vi "Begin.vi"(8 "error in":errorcluster) -> (0 "error out":errorcluster)   [LabVIEW 2014]
doc: "Called before other user functions, this VI is expected to open initial I/O refnums, load in file data, and do all program initialization. Notice that the <B>error out</B> terminal is simply used for data flow. Wiring it to other structures or subVIs ensures that this VI runs first."
uses:
  <vilib>/Rock Robotics/WPI/DriverStation/WPI_DriverStationRobotMode2.ctl
  <vilib>/Rock Robotics/WPI/Joystick/WPI_JoystickDeviceEnum.ctl
  <vilib>/Rock Robotics/SystemInterfaces/DIO/FPGA_DIOPWMChannel.ctl
  <vilib>/Rock Robotics/WPI/Accelerometer/WPI_AccelerometerRange.ctl
  <vilib>/Rock Robotics/SystemInterfaces/AI/FPGA_AIGyroChannel.ctl
  <vilib>/Rock Robotics/WPI/Solenoid/WPI_SolenoidChannel.ctl
  <vilib>/Rock Robotics/SystemInterfaces/DIO/FPGA_DIOChannel.ctl
  <vilib>/Rock Robotics/WPI/Encoder/WPI_EncoderType.ctl
  <vilib>/Rock Robotics/SystemInterfaces/DIO/FPGA_DIORelayChannel.ctl
  Support Files/Robot Global Data.vi
  <vilib>/Rock Robotics/Network Tables/SD Write String Array.vi
  <vilib>/Rock Robotics/WPI/MotorControl/WPI_MotorControlOpen Talon.vi
  <vilib>/Rock Robotics/WPI/Accelerometer/InternalAccelerometer/WPI_AccelerometerInternalOpen.vi
  <vilib>/Rock Robotics/WPI/Solenoid/WPI_SolenoidOpenDouble.vi
  <vilib>/Rock Robotics/WPI/Counter/WPI_CounterDigitalInputToDigitalSource.vi
  <vilib>/Rock Robotics/WPI/Switch/WPI_SwitchOpenLimit.vi
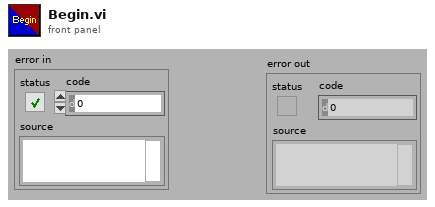
[diagram p1: front panel]
types:
  T1 = typedef "FPGA_DIORelayChannel.ctl" = enum8{"Relay 0", "Relay 1", "Relay 2", "Relay 3", "Invalid"}
  T2 = typedef "FPGA_DIOChannel.ctl" = enum8{"DIO 0", "DIO 1", "DIO 2", "DIO 3", "DIO 4", "DIO 5", "DIO 6", "DIO 7", "DIO 8", "DIO 9", "DIO MXP 0", "DIO MXP 1", "DIO MXP 2", "DIO MXP 3", "DIO MXP 4", "DIO MXP 5", "DIO MXP 6", "DIO MXP 7", "DIO MXP 8", "DIO MXP 9", "DIO MXP 10", "DIO MXP 11", "DIO MXP 12", "DIO MXP 13", "DIO MXP 14", "DIO MXP 15", "Invalid"}
  T3 = typedef "WPI_EncoderType.ctl" = enum16{"1x", "2x", "4x"}
  T4 = typedef "WPI_SolenoidChannel.ctl" = enum8{"Solenoid 0", "Solenoid 1", "Solenoid 2", "Solenoid 3", "Solenoid 4", "Solenoid 5", "Solenoid 6", "Solenoid 7", "Invalid"}
  T5 = typedef "FPGA_DIOPWMChannel.ctl" = enum8{"PWM 0", "PWM 1", "PWM 2", "PWM 3", "PWM 4", "PWM 5", "PWM 6", "PWM 7", "PWM 8", "PWM 9", "PWM MXP 0", "PWM MXP 1", "PWM MXP 2", "PWM MXP 3", "PWM MXP 4", "PWM MXP 5", "PWM MXP 6", "PWM MXP 7", "PWM MXP 8", "PWM MXP 9", "Invalid"}
  T6 = typedef "FPGA_AIGyroChannel.ctl" = enum8{"AI 0", "AI 1", "Invalid"}
  T7 = typedef "WPI_AccelerometerRange.ctl" = enum16{"+/- 2 g", "+/- 4 g", "+/- 8 g"}
  T8 = typedef "WPI_JoystickDeviceEnum.ctl" = enum16{"USB 0", "USB 1", "USB 2", "USB 3", "USB 4", "USB 5"}
  T9 = typedef "WPI_DriverStationRobotMode2.ctl" = enum16{"Autonomous Disabled", "Autonomous Enabled", "Teleop Disabled", "Teleop Enabled", "Disconnected", "Finish", "Test Disabled", "Test Enabled", "Emergency Stopped"}
  T10 = typedef "WPI_JoystickDevRef.ctl" = cluster{"Device":T8}
  T11 = typedef "WPI_SwitchDevRef.ctl" = cluster{"DevStatus":errorcluster, "DIO Channel":T2, "Controller":T12, "CntIndex":T13, "Normally Closed":bool}
  T12 = typedef "FPGA_TypedefDigitalModule.ctl" = enum16{"Controller 1"}
  T13 = typedef "FPGA_CounterCtrSystemIndex.ctl" = enum8{"Ctr 0", "Ctr 1", "Ctr 2", "Ctr 3", "Ctr 4", "Ctr 5", "Ctr 6", "Ctr 7", "Invalid"}
  T14 = typedef "WPI_RelayDevRef.ctl" = cluster{"DevStatus":errorcluster, "Relay Channel":T1, "Controller":T12, "Relay Direction":T15}
  T15 = typedef "WPI_RelayDirection.ctl" = enum16{"Both directions", "Forward only", "Reverse only"}
  T16 = typedef "WPI_MotorControlDeviceRef.ctl" = cluster{"DeviceStatus":errorcluster, "Type":T17, "PWM":cluster{"Controller":T12, "PWM Channel":T5, "DeadBand":T18}, "CAN":cluster{"Device Number":u8, "Control Mode":T19, "Semaphore":T20, "Max Vout":dbl, "TalonSRX Control Mode":T21}, "Invert":bool, "TransformRef":T22, "InvTransformRef":T22}
  T17 = typedef "WPI_MotorControlType.ctl" = enum16{"PWM", "CAN", "CANTalonSRX"}
  T18 = typedef "WPI_PWMDeadband.ctl" = cluster{"Name":string, "maxPositivePwm":i32, "minPositivePwm":i32, "centerPwm":i32, "maxNegativePwm":i32, "minNegativePwm":i32, "angularRange":u16}
  T19 = typedef "WPI_CANJaguar_ControlMode.ctl" = enum8{"Percent VBus", "Current", "Speed", "Position", "Voltage"}
  T20 = typedef "Semaphore RefNum" = refnum<k1>
  T21 = typedef "WPI_CANTalonSRX_APIControlMode.ctl" = enum8{"Percent VBus", "Speed", "Position", "Slave", "Unchanged / Invalid"}
  T22 = typedef "WPI_PWMTransform_ConPane.ctl" = refnum<vi>
  T23 = typedef "WPI_GyroDevRef.ctl" = cluster{"DevStatus":errorcluster, "Analog Module":T24, "Analog Channel":T25, "Offset":dbl, "Gain (VoltsPerDegree/Second)":dbl}
  T24 = typedef "FPGA_TypedefAnalogModule.ctl" = enum16{"Controller 1"}
  T25 = typedef "FPGA_AIChannel.ctl" = enum8{"AI 0", "AI 1", "AI 2", "AI 3", "AI MXP 0", "AI MXP 1", "AI MXP 2", "AI MXP 3", "Invalid"}
  T26 = typedef "WPI_AccelerometerDevRef.ctl" = cluster{"DevStatus":errorcluster, "Controller":T24, "Scaling":T27, "Analog Channels":T28, "I2C Bus":T29, "SPI Bus":T30, "Accel Range":T31, "ADXL345 Axes":T32, "Handle":i32, "Device Address":u8, "Accel Type":enum16{"Analog", "ADXL345 I2C", "ADXL345 SPI", "Internal"}}
  T27 = typedef "WPI_AccelerometerScaling.ctl" = cluster{"Gain (VoltsPerG)":dbl, "Center Voltage":dbl}
  T28 = typedef "WPI_AccelerometerAnalogChannels.ctl" = cluster{"X-Axis":T25, "Y-Axis":T25, "Z-Axis":T25}
  T29 = typedef "i2c_bus.ctl" = enum16{"I2C On-Board", "I2C MXP", "Invalid"}
  T30 = typedef "spi_bus.ctl" = enum16{"SPI On-Board, CS0", "SPI On-Board, CS1", "SPI On-Board, CS2", "SPI On-Board, CS3", "SPI MXP", "Invalid"}
  T31 = typedef "ADXL345 Range.ctl" = u8
  T32 = typedef "WPI_AccelerometerADXL345 Axes.ctl" = cluster{"X-Axis":bool, "Y-Axis":bool, "Z-Axis":bool}
  T33 = typedef "WPI_DigitalInputDevRef.ctl" = cluster{"DevStatus":errorcluster, "DIO Channel":T2, "Controller":T12}
  T34 = typedef "FPGA_CounterEncoderSourceConvertionLVSourceType.ctl" = cluster{"DevStatus":errorcluster, "AnalogTriggerMode?":bool, "DigitalMode":cluster{"Controller":T12, "DIO Channel":T35}, "AnalogTriggerMode":cluster{"AnalogTriggerIndex":T36, "OutputType":T37}}
  T35 = typedef "FPGA_DIODigitalSourceChannel.ctl" = enum8{"DIO 0", "DIO 1", "DIO 2", "DIO 3", "DIO 4", "DIO 5", "DIO 6", "DIO 7", "DIO 8", "DIO 9", "DIO MXP 0", "DIO MXP 1", "DIO MXP 2", "DIO MXP 3", "DIO MXP 4", "DIO MXP 5", "DIO MXP 6", "DIO MXP 7", "DIO MXP 8", "DIO MXP 9", "DIO MXP 10", "DIO MXP 11", "DIO MXP 12", "DIO MXP 13", "DIO MXP 14", "DIO MXP 15", "Disabled"}
  T36 = typedef "FPGA_AnalogTriggerIndex.ctl" = enum8{"Trig 0", "Trig 1", "Trig 2", "Trig 3", "Trig 4", "Trig 5", "Trig 6", "Trig 7", "Invalid"}
  T37 = typedef "FPGA_AnalogTriggerOutType.ctl" = enum16{"InWindow", "TriggerState", "Rising", "Falling"}
  T38 = typedef "WPI_EncoderDevRef.ctl" = cluster{"DevStatus":errorcluster, "EncoderIndex":T39, "CounterIndex":T13, "DistancePerCount":dbl, "Decoding Type":T3}
  T39 = typedef "FPGA_EncoderIdx.ctl" = enum8{"Enc 0", "Enc 1", "Enc 2", "Enc 3", "Enc 4", "Enc 5", "Enc 6", "Enc 7", "Invalid"}
  T40 = typedef "WPI_SolenoidDevRef.ctl" = cluster{"DevStatus":errorcluster, "Pneumatics Control Module":u8, "Forward Solenoid Channel":T4, "Reverse Solenoid Channel":T4}
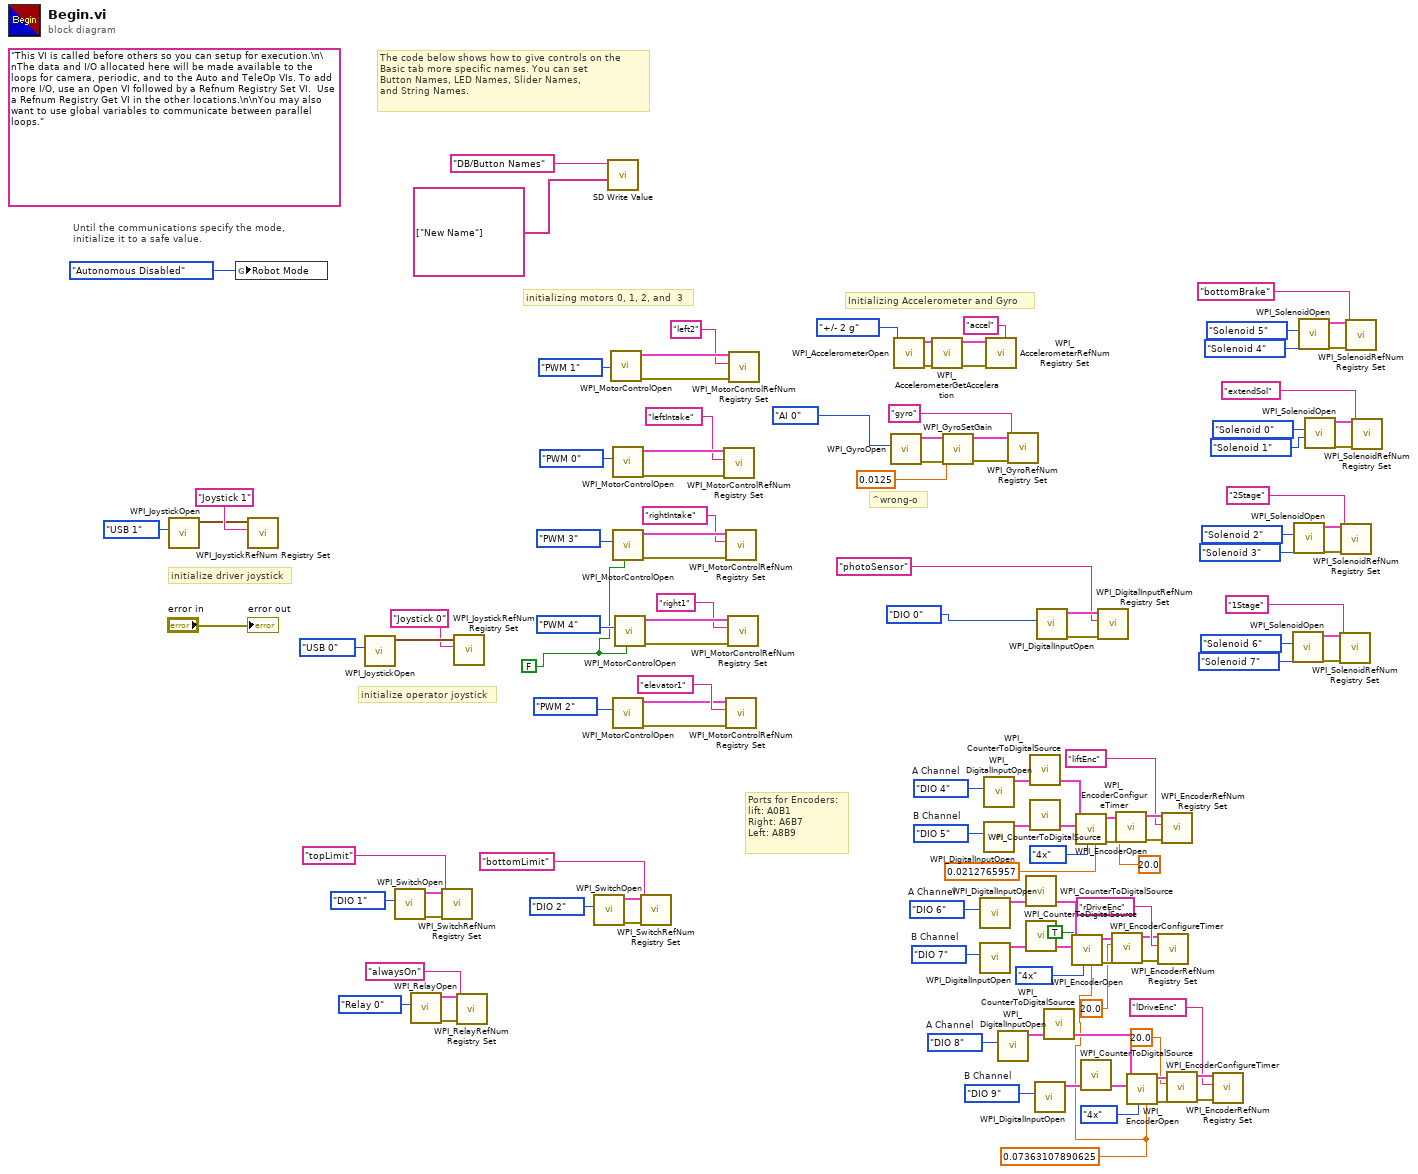
[diagram p0: block diagram]
diagram:
  w13 = 0.07363107890625 ("DistancePerCount")
  w36 = FPGA_DIOChannel."DIO 9"  # B Channel
  w35 = FPGA_DIOChannel."DIO 8"  # A Channel
  w37 = FPGA_DIOChannel."DIO 7"  # B Channel
  w38 = FPGA_DIOChannel."DIO 6"  # A Channel
  w58 = FPGA_DIOChannel."DIO 5"  # B Channel
  w57 = FPGA_DIOChannel."DIO 4"  # A Channel
  w79 = FALSE ("Invert")
  (unwired) "This VI is called before others so you can setup for execution.\n\nThe data and I/O allocated here will be made available to the loops for camera, periodic, and to the Auto and TeleOp VIs. To add more I/O, use an Open VI followed by a Refnum Registry Set VI.  Use a Refnum Registry Get VI in the other locations.\n\nYou may also want to use global variables to communicate between parallel loops."
  # "Ports for Encoders:\nlift: A0B1\nRight: A6B7\nLeft: A8B9"
  # "^wrong-o"
  # "Initializing Accelerometer and Gyro"
  # "initialize operator joystick"
  # "initializing motors 0, 1, 2, and  3"
  # "The code below shows how to give controls on the\nBasic tab more specific names. You can set\nButton Names, LED Names, Slider Names,\nand String Names."
  # "initialize driver joystick"
  # "Until the communications specify the mode,\ninitialize it to a safe value."
  n1 = call <vilib>:"WPI_JoystickOpen.vi"("JoystickDevice"=WPI_JoystickDeviceEnum."USB 1") -> ("JoystickDevRef"=w120:T10)  [unwired: 10 in]
  n2 = global write "Robot Global Data.vi" "Robot Mode"(WPI_DriverStationRobotMode2."Autonomous Disabled" ("Robot Mode")) -> ()
  n3 = call <vilib>:"WPI_JoystickRefNum Registry Set.vi"("refnum name"="Joystick 1", "JoystickDevRef"=w120) -> ()  [unwired: 8 in, 2 out]
  n4 = call <vilib>:"WPI_JoystickOpen.vi"("JoystickDevice"=WPI_JoystickDeviceEnum."USB 0") -> ("JoystickDevRef"=w103:T10)  [unwired: 10 in]
  n5 = call-poly <vilib>:"WPI_SwitchOpen.vi"("DIO Channel"=FPGA_DIOChannel."DIO 1") -> ("error out"=w12:errorcluster, "SwitchDevRef"=w11:T11)  [unwired: 9 in]
  n6 = call <vilib>:"WPI_RelayOpen.vi"("Relay Channel"=FPGA_DIORelayChannel."Relay 0") -> ("error out"=w4:errorcluster, "RelayDevRef"=w3:T14)  [unwired: 9 in]
  n7 = call <vilib>:"WPI_SwitchRefNum Registry Set.vi"("error in (no error)"=w12, "refnum name"="topLimit", "SwitchDevRef"=w11) -> ()  [unwired: 7 in, 2 out]
  n8 = call <vilib>:"WPI_JoystickRefNum Registry Set.vi"("refnum name"="Joystick 0", "JoystickDevRef"=w103) -> ()  [unwired: 8 in, 2 out]
  n9 = call <vilib>:"WPI_RelayRefNum Registry Set.vi"("error in (no error)"=w4, "refnum name"="alwaysOn", "RelayDevRef"=w3) -> ()  [unwired: 7 in, 2 out]
  n10 = call-poly <vilib>:"WPI_SwitchOpen.vi"("DIO Channel"=FPGA_DIOChannel."DIO 2") -> ("error out"=w5:errorcluster, "SwitchDevRef"=w6:T11)  [unwired: 9 in]
  n11 = call-poly <vilib>:"SD Write Value.vi"("String Array"=string[] ["New Name"], "Name"="DB/Button Names") -> ()  [unwired: 8 in, 2 out]
  n12 = call-poly <vilib>:"WPI_MotorControlOpen.vi"("PWM Channel"=FPGA_DIOPWMChannel."PWM 1") -> ("error out"=w99:errorcluster, "MotorControlDeviceRef"=w100:T16)  [unwired: 9 in]
  n13 = call-poly <vilib>:"WPI_MotorControlOpen.vi"("PWM Channel"=FPGA_DIOPWMChannel."PWM 0") -> ("error out"=w109:errorcluster, "MotorControlDeviceRef"=w115:T16)  [unwired: 9 in]
  n14 = call-poly <vilib>:"WPI_MotorControlOpen.vi"("Invert"=w79, "PWM Channel"=FPGA_DIOPWMChannel."PWM 3") -> ("error out"=w104:errorcluster, "MotorControlDeviceRef"=w114:T16)  [unwired: 8 in]
  n15 = call-poly <vilib>:"WPI_MotorControlOpen.vi"("PWM Channel"=FPGA_DIOPWMChannel."PWM 2") -> ("error out"=w83:errorcluster, "MotorControlDeviceRef"=w80:T16)  [unwired: 9 in]
  n16 = call-poly <vilib>:"WPI_MotorControlOpen.vi"("Invert"=w79, "PWM Channel"=FPGA_DIOPWMChannel."PWM 4") -> ("error out"=w105:errorcluster, "MotorControlDeviceRef"=w113:T16)  [unwired: 8 in]
  n17 = call <vilib>:"WPI_SwitchRefNum Registry Set.vi"("error in (no error)"=w5, "refnum name"="bottomLimit", "SwitchDevRef"=w6) -> ()  [unwired: 7 in, 2 out]
  n18 = call <vilib>:"WPI_MotorControlRefNum Registry Set.vi"("error in (no error)"=w109, "refnum name"="leftIntake", "MotorControlDevRef"=w115) -> ()  [unwired: 7 in, 2 out]
  n19 = call <vilib>:"WPI_MotorControlRefNum Registry Set.vi"("error in (no error)"=w104, "refnum name"="rightIntake", "MotorControlDevRef"=w114) -> ()  [unwired: 7 in, 2 out]
  n20 = call <vilib>:"WPI_MotorControlRefNum Registry Set.vi"("error in (no error)"=w83, "refnum name"="elevator1", "MotorControlDevRef"=w80) -> ()  [unwired: 7 in, 2 out]
  n21 = call <vilib>:"WPI_MotorControlRefNum Registry Set.vi"("error in (no error)"=w105, "refnum name"="right1", "MotorControlDevRef"=w113) -> ()  [unwired: 7 in, 2 out]
  n22 = call <vilib>:"WPI_MotorControlRefNum Registry Set.vi"("error in (no error)"=w99, "refnum name"="left2", "MotorControlDevRef"=w100) -> ()  [unwired: 7 in, 2 out]
  n23 = call <vilib>:"WPI_GyroOpen.vi"("Analog Channel"=FPGA_AIGyroChannel."AI 0") -> ("error out"=w85:errorcluster, "GyroDevRef"=w88:T23)  [unwired: 8 in, 1 out]
  n24 = call-poly <vilib>:"WPI_AccelerometerOpen.vi"("Accel Range"=WPI_AccelerometerRange."+/- 2 g") -> ("error out"=w94:errorcluster, "AccelerometerDevRef"=w95:T26)  [unwired: 9 in]
  n25 = call <vilib>:"WPI_AccelerometerGetAcceleration.vi"("error in"=w94, "AccelerometerDevRef"=w95) -> ("error out"=w91:errorcluster, "AccelerometerDevRef"=w93:T26)  [unwired: 7 in, 1 out]
  n26 = call <vilib>:"WPI_GyroSetGain.vi"("error in (no error)"=w85, "Gain (VoltsPerDegree/Second)"=0.0125, "GyroDevRef"=w88) -> ("error out"=w86:errorcluster, "GyroDevRef"=w87:T23)  [unwired: 7 in]
  n27 = call <vilib>:"WPI_DigitalInputOpen.vi"("DIO Channel"=w38) -> ("DigitalInputDevRef"=w41:T33)  [unwired: 2 in, 8 out]
  n28 = call <vilib>:"WPI_DigitalInputOpen.vi"("DIO Channel"=w37) -> ("DigitalInputDevRef"=w40:T33)  [unwired: 2 in, 8 out]
  n29 = call <vilib>:"WPI_DigitalInputOpen.vi"("DIO Channel"=w57) -> ("DigitalInputDevRef"=w54:T33)  [unwired: 2 in, 8 out]
  n30 = call <vilib>:"WPI_DigitalInputOpen.vi"("DIO Channel"=w58) -> ("DigitalInputDevRef"=w55:T33)  [unwired: 2 in, 8 out]
  n31 = call <vilib>:"WPI_AccelerometerRefNum Registry Set.vi"("error in (no error)"=w91, "refnum name"="accel", "AccelerometerDevRef"=w93) -> ()  [unwired: 7 in, 2 out]
  n32 = call <vilib>:"WPI_DigitalInputOpen.vi"("DIO Channel"=w35) -> ("DigitalInputDevRef"=w32:T33)  [unwired: 2 in, 8 out]
  n33 = call <vilib>:"WPI_GyroRefNum Registry Set.vi"("error in (no error)"=w86, "refnum name"="gyro", "GyroDevRef"=w87) -> ()  [unwired: 7 in, 2 out]
  n34 = call-poly <vilib>:"WPI_CounterToDigitalSource.vi"("DigitalInputDevRef"=w41) -> ("Digital Source"=w42:T34)  [unwired: 6 out]
  n35 = call-poly <vilib>:"WPI_CounterToDigitalSource.vi"("DigitalInputDevRef"=w40) -> ("Digital Source"=w39:T34)  [unwired: 6 out]
  n36 = call-poly <vilib>:"WPI_CounterToDigitalSource.vi"("DigitalInputDevRef"=w54) -> ("Digital Source"=w53:T34)  [unwired: 6 out]
  n37 = call-poly <vilib>:"WPI_CounterToDigitalSource.vi"("DigitalInputDevRef"=w55) -> ("Digital Source"=w56:T34)  [unwired: 6 out]
  n38 = call <vilib>:"WPI_DigitalInputOpen.vi"("DIO Channel"=w36) -> ("DigitalInputDevRef"=w33:T33)  [unwired: 2 in, 8 out]
  n39 = call <vilib>:"WPI_DigitalInputOpen.vi"("DIO Channel"=FPGA_DIOChannel."DIO 0") -> ("error out"=w17:errorcluster, "DigitalInputDevRef"=w18:T33)  [unwired: 9 in]
  n40 = call-poly <vilib>:"WPI_CounterToDigitalSource.vi"("DigitalInputDevRef"=w32) -> ("Digital Source"=w31:T34)  [unwired: 6 out]
  n41 = call <vilib>:"WPI_EncoderOpen.vi"("DistancePerCount"=w13, "Decoding Type"=WPI_EncoderType."4x", "Invert Direction (False)"=TRUE, "BSource"=w39, "ASource"=w42) -> ("error out"=w43:errorcluster, "EncoderDevRef"=w44:T38)  [unwired: 3 in, 2 out]
  n42 = call <vilib>:"WPI_EncoderOpen.vi"("DistancePerCount"=0.0212765957, "Decoding Type"=WPI_EncoderType."4x", "BSource"=w56, "ASource"=w53) -> ("error out"=w52:errorcluster, "EncoderDevRef"=w51:T38)  [unwired: 4 in, 2 out]
  n43 = call-poly <vilib>:"WPI_CounterToDigitalSource.vi"("DigitalInputDevRef"=w33) -> ("Digital Source"=w34:T34)  [unwired: 6 out]
  n44 = call <vilib>:"WPI_DigitalInputRefNum Registry Set.vi"("error in (no error)"=w17, "refnum name"="photoSensor", "DigitalInputDevRef"=w18) -> ()  [unwired: 7 in, 2 out]
  n45 = call <vilib>:"WPI_EncoderConfigureTimer.vi"("error in (no error)"=w43, "Minimum Rate"=20.0, "EncoderDevRef"=w44) -> ("error out"=w45:errorcluster, "EncoderDevRef"=w46:T38)  [unwired: 7 in]
  n46 = call <vilib>:"WPI_EncoderConfigureTimer.vi"("error in (no error)"=w52, "Minimum Rate"=20.0, "EncoderDevRef"=w51) -> ("error out"=w50:errorcluster, "EncoderDevRef"=w49:T38)  [unwired: 7 in]
  n47 = call <vilib>:"WPI_EncoderOpen.vi"("DistancePerCount"=w13, "Decoding Type"=WPI_EncoderType."4x", "BSource"=w34, "ASource"=w31) -> ("error out"=w30:errorcluster, "EncoderDevRef"=w29:T38)  [unwired: 4 in, 2 out]
  n48 = call <vilib>:"WPI_EncoderRefNum Registry Set.vi"("error in (no error)"=w45, "refnum name"="rDriveEnc", "EncoderDevRef"=w46) -> ()  [unwired: 7 in, 2 out]
  n49 = call <vilib>:"WPI_EncoderRefNum Registry Set.vi"("error in (no error)"=w50, "refnum name"="liftEnc", "EncoderDevRef"=w49) -> ()  [unwired: 7 in, 2 out]
  n50 = call <vilib>:"WPI_EncoderConfigureTimer.vi"("error in (no error)"=w30, "Minimum Rate"=20.0, "EncoderDevRef"=w29) -> ("error out"=w28:errorcluster, "EncoderDevRef"=w27:T38)  [unwired: 7 in]
  n51 = call <vilib>:"WPI_EncoderRefNum Registry Set.vi"("error in (no error)"=w28, "refnum name"="lDriveEnc", "EncoderDevRef"=w27) -> ()  [unwired: 7 in, 2 out]
  n52 = call-poly <vilib>:"WPI_SolenoidOpen.vi"("Reverse Solenoid Channel"=WPI_SolenoidChannel."Solenoid 7", "Forward Solenoid Channel"=WPI_SolenoidChannel."Solenoid 6" ("Solenoid Channel")) -> ("error out"=w60:errorcluster, "SolenoidDevRef"=w59:T40)  [unwired: 8 in]
  n53 = call-poly <vilib>:"WPI_SolenoidOpen.vi"("Reverse Solenoid Channel"=WPI_SolenoidChannel."Solenoid 3", "Forward Solenoid Channel"=WPI_SolenoidChannel."Solenoid 2" ("Solenoid Channel")) -> ("error out"=w67:errorcluster, "SolenoidDevRef"=w68:T40)  [unwired: 8 in]
  n54 = call-poly <vilib>:"WPI_SolenoidOpen.vi"("Reverse Solenoid Channel"=WPI_SolenoidChannel."Solenoid 4", "Forward Solenoid Channel"=WPI_SolenoidChannel."Solenoid 5" ("Solenoid Channel")) -> ("error out"=w77:errorcluster, "SolenoidDevRef"=w78:T40)  [unwired: 8 in]
  n55 = call-poly <vilib>:"WPI_SolenoidOpen.vi"("Reverse Solenoid Channel"=WPI_SolenoidChannel."Solenoid 1", "Forward Solenoid Channel"=WPI_SolenoidChannel."Solenoid 0" ("Solenoid Channel")) -> ("error out"=w70:errorcluster, "SolenoidDevRef"=w69:T40)  [unwired: 8 in]
  n56 = call <vilib>:"WPI_SolenoidRefNum Registry Set.vi"("error in (no error)"=w60, "refnum name"="1Stage", "SolenoidDevRef"=w59) -> ()  [unwired: 7 in, 2 out]
  n57 = call <vilib>:"WPI_SolenoidRefNum Registry Set.vi"("error in (no error)"=w67, "refnum name"="2Stage", "SolenoidDevRef"=w68) -> ()  [unwired: 7 in, 2 out]
  n58 = call <vilib>:"WPI_SolenoidRefNum Registry Set.vi"("error in (no error)"=w77, "refnum name"="bottomBrake", "SolenoidDevRef"=w78) -> ()  [unwired: 7 in, 2 out]
  n59 = call <vilib>:"WPI_SolenoidRefNum Registry Set.vi"("error in (no error)"=w70, "refnum name"="extendSol", "SolenoidDevRef"=w69) -> ()  [unwired: 7 in, 2 out]
  "error out" <- "error in"
